vi "FFT.vi"() -> ()   [LabVIEW 2020]
uses:
  <vilib>/rvi/Analysis/measure/FFT/simModelSupport/niFPGA FFT Outside SCTL Sim Properties.ctl
  <vilib>/rvi/Analysis/measure/FFT/simModelSupport/niFPGA FFT Sim Types.ctl
  <vilib>/rvi/Analysis/measure/FFT/simModelSupport/niFpgaFFTSimArithmeticProperties.ctl
  <vilib>/rvi/Analysis/measure/FFT/simModelSupport/niFpgaFFTSimDfxp.ctl
  <vilib>/fxp/LVFixedPointQuantizationPolicyTypeDef.ctl
  <vilib>/rvi/Emulation/niFpgaGetClockAttributes.vi
  <vilib>/rvi/Emulation/niFpgaSctlEmulationGetInTimedLoop.vi
  <vilib>/rvi/Emulation/niFpgaEmulationReportErrorSimple.vi
  <vilib>/rvi/interface/RandomDataEmulation/niFpgaRandomDataHandleErrors.vi
  <vilib>/rvi/Analysis/measure/FFT/simModelSupport/niFpgaFFTSimModelOutsideSCTLCore.vi
  <vilib>/rvi/Emulation/niFpgaCriticalErrorInLSC.vi
  <vilib>/rvi/DataTransferAndStorage/Container/XNode/niFpgaContainer.xnode
  <vilib>/rvi/interface/RandomDataEmulation/nirviRandomDataFpgaReadWriteTemplate.vi
  <vilib>/rvi/Analysis/measure/FFT/XNode/niFpgaFFT.xnode
panel:
  out "data index":u16
  out "x-y (microsecond)":u32
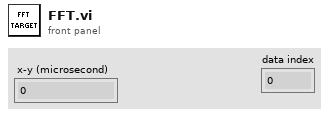
[diagram p1: front panel]
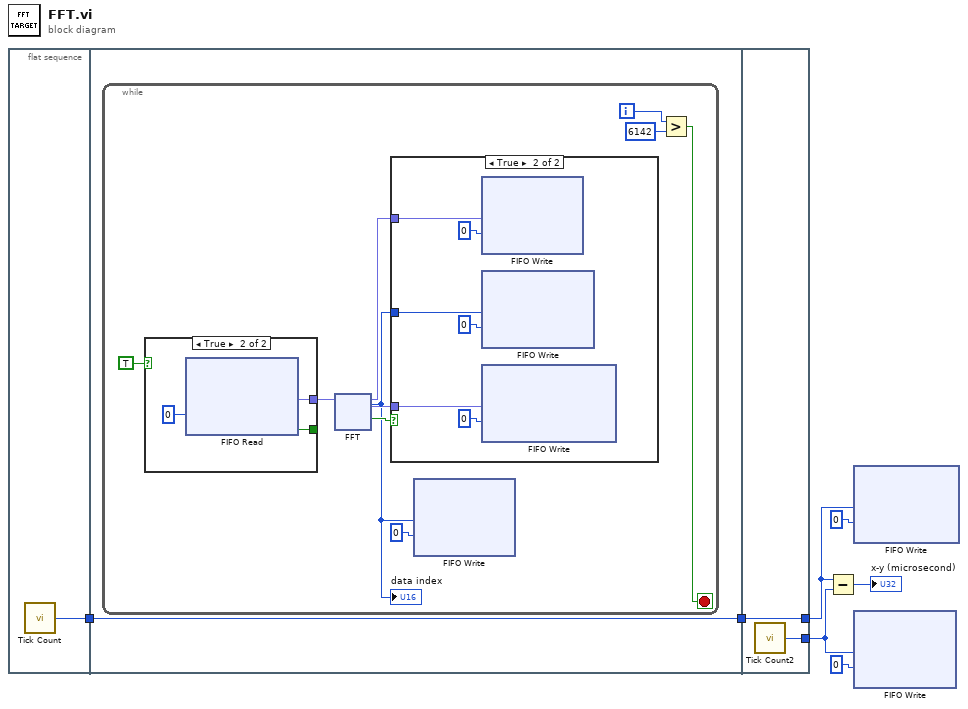
[diagram p0: block diagram]
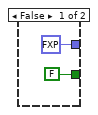
[diagram p2: hidden frame]
diagram:
  n1 = flat-sequence {
    tunnel: [w8] -> w7
    tunnel: [w9] -> w6
    tunnel: w7 -> [w9]
    tunnel: [w52] -> w4
    tunnel: w6 -> [w52]
    tunnel: [w51] -> w3
    frame #0 {
      n2 = call "Tick Count"() -> ("Tick Count(uSec)"=w8:u32)
    }
    frame #1 {
      n3 = while {
        i -> [w15]
        stop <- w16 stop-if-true
        n4 = case shown="True" TRUE ("ready for input") {
          tunnel: [fxp<+/-,24,7> 0.0 ("Element") w24] -> w19
          tunnel: [FALSE ("Timed Out?") w22] -> _
          frame False {
          }
          frame True {
            n5 = xnode ("FIFO Read")("Timeout"=0) -> ("Element"=w24:fxp<+/-,24,7>, "Timed Out?"=w22:bool)  [unwired: 1 in, 1 out]
          }
        }
        n6 = xnode ("FFT")("real data in"=w19) -> ("data index"=w11:u16, "real data out"=w13:fxp<+/-,32,16>, "imaginary data out"=w12:fxp<+/-,32,16>, "output valid"=w17:bool)  [unwired: 2 in]
        "data index" <- w11
        n7 = case shown="True" w17 {
          tunnel: w12 -> [_ w25]
          tunnel: w13 -> [_ w26]
          tunnel: w11 -> [_ w28]
          frame False {
          }
          frame True {
            n8 = xnode ("FIFO Write")("Element"=w26, "Timeout"=0) -> ()  [unwired: 1 in, 2 out]
            n9 = xnode ("FIFO Write")("Element"=w28, "Timeout"=0) -> ()  [unwired: 1 in, 2 out]
            n10 = xnode ("FIFO Write")("Element"=w25, "Timeout"=0) -> ()  [unwired: 1 in, 2 out]
          }
        }
        n11 = xnode ("FIFO Write")("Element"=w11, "Timeout"=0) -> ()  [unwired: 1 in, 2 out]
        n12 = Greater?(x=w15, y=6142 ("Timeout")) -> (0:w16:bool)
      }
    }
    frame #2 {
      n13 = call "Tick Count2"() -> ("Tick Count(uSec)"=w51:u32)
    }
  }
  n14 = Subtract(x=w4, y=w3) -> (x-y=→"x-y (microsecond)":u32)
  n15 = xnode ("FIFO Write")("Element"=w4, "Timeout"=0) -> ()  [unwired: 1 in, 2 out]
  n16 = xnode ("FIFO Write")("Element"=w3, "Timeout"=0) -> ()  [unwired: 1 in, 2 out]
